vi "FTW-Endpoint-Multipart-Send.vi"(0 "FTW Endpoint":refnum<class "FTW-Endpoint.lvclass">, 5 "Multipart Message":string[](array[string]), 7 "Timeout":i32 format="%dmsec", 11 "error in":errorcluster) -> (4 "FTW Endpoint out":refnum<class "FTW-Endpoint.lvclass">, 6 "Timed out?":bool, 15 "error out":errorcluster)   [LabVIEW 2013, in "FTW-Endpoint.lvclass"]
uses:
  FTW-Endpoint.lvclass
  FTW-Endpoint.lvclass/FTW-Endpoint.ctl
panel:
  # "Inputs"
  # "Outputs"
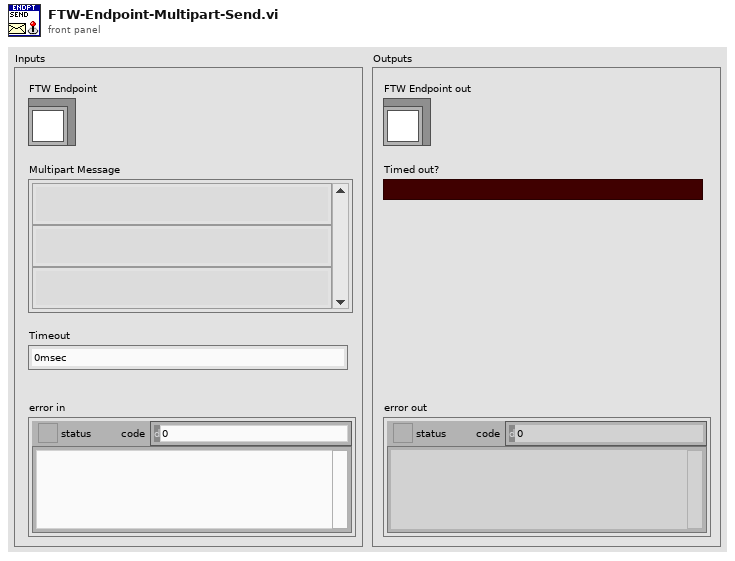
[diagram p1: front panel]
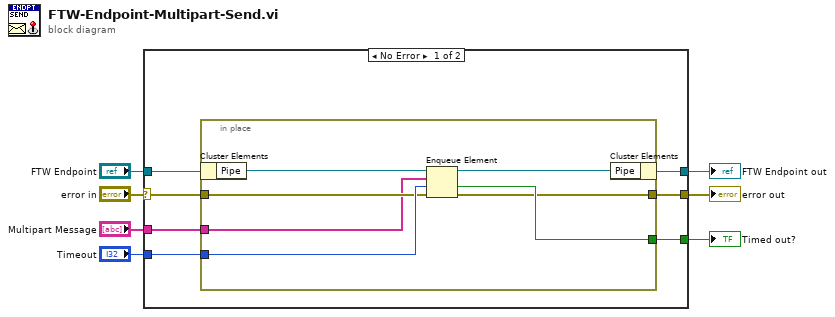
[diagram p0: block diagram]
diagram:
  n1 = case shown="No Error" "error in" {
    selector: "error in" -> [w12 w23]
    tunnel: [w11 w23] -> w7
    tunnel: [w8 w22] -> w5
    tunnel: "FTW Endpoint" -> [w9 w22]
    tunnel: "Multipart Message" -> [w10 _]
    tunnel: [w14 _] -> w2
    tunnel: "Timeout" -> [w13 _]
    frame No Error {
      n2 = in-place {
        in-place-border: [w21] -> w14
        in-place-border: w13 -> [w20]
        in-place-border: w12 -> [w19]
        in-place-border: [w18] -> w11
        in-place-border: w10 -> [w17]
        n3 = in-place-cluster #1(w9) -> ("Pipe"=w16:refnum<queue>)
        n4 = Enqueue Element(queue=w16, element=w17, timeout in ms (-1)=w20, error in (no error)=w19) -> (queue out=w15:refnum<queue>, timed out?=w21:bool, error out=w18:errorcluster)
        n5 = in-place-cluster #1("Pipe"=w15) -> (w8:refnum<class "FTW-Endpoint.lvclass">)
      }
    }
    frame Error {
    }
  }
  "error out" <- w7
  "FTW Endpoint out" <- w5
  "Timed out?" <- w2
